vi "solar_excel Cell Values (Row).vi"(11 "Cells in":string[][](array[string])) -> (3 "Values":string[][](array[string]), 5 "Row Headers":string[](array[string]))   [LabVIEW 2018]
doc: "This removes the Row Headers (first column)."
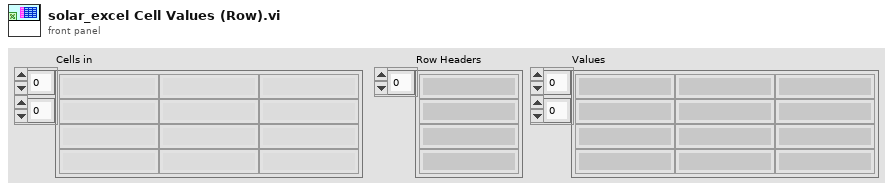
[diagram p1: front panel]
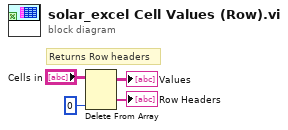
[diagram p0: block diagram]
diagram:
  # "Returns Row headers"
  n1 = Delete From Array(array="Cells in", index (col)=0 ("disabled index (col)")) -> (deleted portion=→"Row Headers":string[], array with subset deleted=→"Values":string[][])  [unwired: 2 in]
